vi "week08_Ex01.vi"() -> ()   [LabVIEW 2017]
panel:
  out "Array":u8[](array[numeric])
  out "i":i32
  out "ตัวเลขที่สุ่มได้ 10 เลข":u8[](array[numeric])
  out "0-100":u8
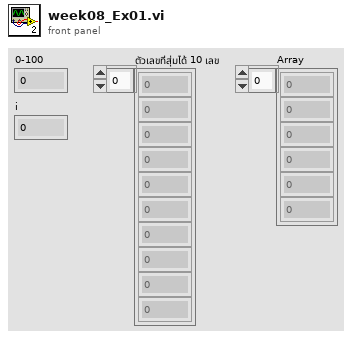
[diagram p1: front panel]
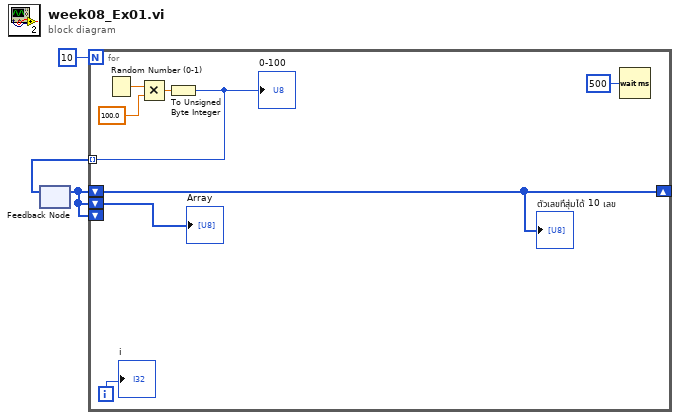
[diagram p0: block diagram]
diagram:
  n1 = feedback #1() -> (w1:u8[])  [unwired: 1 in]
  n2 = for {
    N: 10 -> [_]
    shift-right: [w5] -> _
    shift-left: w1 -> [w5]
    tunnel: [w7] -> w2 mode=indexing
    shift-left: w1 -> [w4]
    shift-left: w1 -> [_]
    i -> [w6]
    n3 = Random Number (0-1)() -> (number: 0 to 1=w9:dbl)
    n4 = Multiply(x=w9, y=100.0) -> (x*y=w10:dbl)
    n5 = To Unsigned Byte Integer(number=w10) -> (unsigned 8bit integer=w7:u8)
    "0-100" <- w7
    n6 = Wait (ms)(milliseconds to wait=u32 500) -> ()  [unwired: 1 out]
    "ตัวเลขที่สุ่มได้ 10 เลข" <- w5
    "i" <- w6
    "Array" <- w4
  }
  n7 = feedback-in #1(w2) -> ()
